vi "PathPlanner_GoalEndState_Flip.vi"(11 "GoalEndState":T1={"VelocityMPS"=0.0, "Rotation"={"VALUE"=0.0, "COS"=1.0, "SIN"=0.0}} {"Rotation"."SIN" format="%13.4f"; "Rotation"."COS" format="%13.4f"; "Rotation"."VALUE" format="%13.4f"}) -> (3 "FlippedGoalEndState":T1={"VelocityMPS"=0.0, "Rotation"={"VALUE"=0.0, "COS"=1.0, "SIN"=0.0}} {"Rotation"."SIN" format="%13.4f"; "Rotation"."COS" format="%13.4f"; "Rotation"."VALUE" format="%13.4f"})   [LabVIEW 2019, in "PathPlanner24.lvlib"]
doc: "Flip the goal end state for the other side of the field, maintaining a blue alliance origin\n \n\nInputs: \n -- GoalEndState - cluster - definition data structure\n\nOutputs:\n -- FlippedGoalEndState - cluster - The flipped end state"
uses:
  TypeDef/PathPlannerGoalEndState.ctl
  <vilib>/Rock Robotics/WPI/ThirdParty/JAS_Junk/TrajLib/TypeDef/ROTATION2D.ctl
  PathPlanner24.lvlib
  <vilib>/Rock Robotics/WPI/ThirdParty/JAS_Junk/TrajLib/Trajectory_Library.lvlib
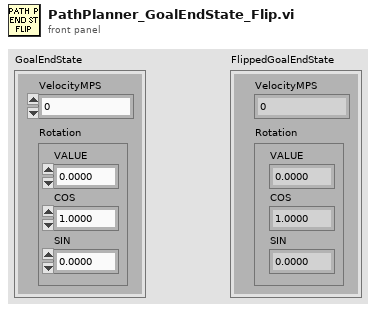
[diagram p1: front panel]
types:
  T1 = typedef "PathPlanner24.lvlib/PathPlannerGoalEndState.ctl" = cluster{"VelocityMPS":dbl, "Rotation":T2}
  T2 = typedef "Trajectory_Library.lvlib/ROTATION2D.ctl" = cluster{"VALUE":dbl, "COS":dbl, "SIN":dbl}
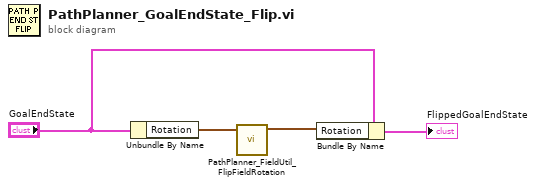
[diagram p0: block diagram]
diagram:
  n1 = Unbundle By Name("GoalEndState") -> ("Rotation"=w2:T2)
  n2 = call "PathPlanner_FieldUtil_FlipFieldRotation.vi"("rotation"=w2) -> ("flippedRotation"=w1:T2)  [unwired: 10 in]
  n3 = Bundle By Name(cluster="GoalEndState", "Rotation"=w1) -> (→"FlippedGoalEndState":T1)
